vi "Run Action.vi"(8 "error in (no error)":errorcluster, 10 "Package":refnum<class "PackageAbstract.lvclass">, 11 "InstallAction in":refnum<class "InstallAction.lvclass">) -> (0 "error out":errorcluster, 2 "Problems":string[](array[string]), 3 "InstallAction out":refnum<class "InstallAction.lvclass">)   [LabVIEW 2020, in "GPackTools.lvlib" / "InstallAction.lvclass"]
uses:
  InstallAction.lvclass
  GPack/PackageAbstract/PackageAbstract.lvclass
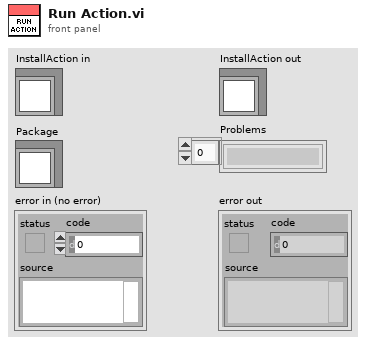
[diagram p1: front panel]
types:
  T1 = typedef "GPack.lvlib/Dependency.ctl" = cluster{"Info":T2, "Path":path}
  T2 = typedef "GPack.lvlib/Package Info.ctl" = cluster{"Name":string, "Type":string, "Host":string, "Path":string, "Branch":string, "Version":string}
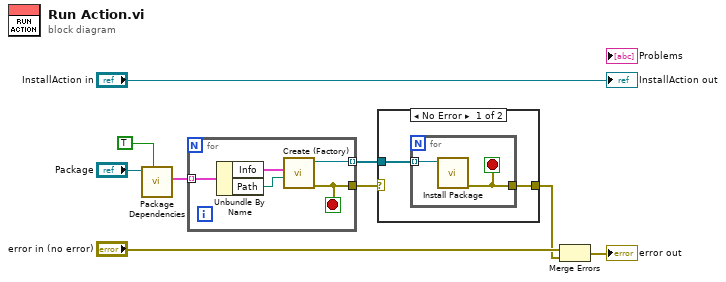
[diagram p0: block diagram]
diagram:
  n1 = call-dynamic "Package Dependencies.vi"("Absolute Path (F)"=TRUE, "PackageAbstract in"="Package") -> ("Dependencies"=w6:T1[])  [unwired: 8 in, 1 out]
  n2 = for {
    tunnel: w6 -> [w14] mode=indexing
    tunnel: [w11] -> w5
    tunnel: [w10] -> w4 mode=indexing
    stop <- w11 stop-if-true
    n3 = Unbundle By Name(w14) -> ("Info"=w13:T2, "Path"=w12:path)
    n4 = call "Create (Factory).vi"("Folder"=w12, "Package Info"=w13) -> ("error out"=w11:errorcluster, "PackageAbstract out"=w10:refnum<class "PackageAbstract.lvclass">)  [unwired: 8 in]
  }
  n5 = case shown="No Error" w5 {
    selector: w5 -> [_ w19]
    tunnel: w4 -> [w16 _]
    tunnel: [w15 w19] -> w2
    frame No Error {
      n6 = for {
        tunnel: w16 -> [w18] mode=indexing
        tunnel: [w17] -> w15
        stop <- w17 stop-if-true
        n7 = call-dynamic "Install Package.vi"("Package in"=w18) -> ("error out"=w17:errorcluster)  [unwired: 9 in, 1 out]
      }
    }
    frame Error {
    }
  }
  n8 = Merge Errors("error in (no error)", w2) -> (→"error out":errorcluster)
  "InstallAction out" <- "InstallAction in"
